vi "ClearPortList.vi"(1 "topic port":u16) -> ()   [LabVIEW 2012]
doc: "Clears a port from the server port list"
uses:
  <userlib>/ROSforLV/ROS/Code/_ROSDefinition.vi
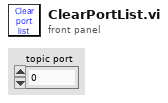
[diagram p1: front panel]
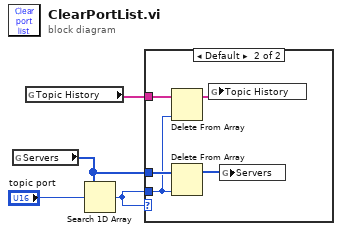
[diagram p0: block diagram]
diagram:
  n1 = global read "_ROSDefinition.vi" "Servers"() -> (w3:u16[])
  n2 = global read "_ROSDefinition.vi" "Topic History"() -> (w1:string[])
  n3 = Search 1D Array(1D array=w3, element="topic port") -> (index of element=w2:i32)  [unwired: 1 in]
  n4 = case shown="Default" w2 {
    tunnel: w2 -> [_ w7]
    tunnel: w3 -> [_ w9]
    tunnel: w1 -> [_ w6]
    frame -1 {
    }
    frame Default {
      n5 = Delete From Array(array=w6, index=w7) -> (array with subset deleted=w5:string[])  [unwired: 1 in, 1 out]
      n6 = Delete From Array(array=w9, index=w7) -> (array with subset deleted=w8:u16[])  [unwired: 1 in, 1 out]
      n7 = global write "_ROSDefinition.vi" "Topic History"(w5) -> ()
      n8 = global write "_ROSDefinition.vi" "Servers"(w8) -> ()
    }
  }
